vi "Menu Button - Load Config File.vi"(8 "error in (no error)":errorcluster, 11 "Path":path=path "C:/Projects/Trackside-CrawlerFinalDriveTestStand/Codeline/Main Codeline/Software/Config Files_Host/MenuConfig.ini") -> (0 "error out":errorcluster, 1 "Button[]":string[](array[string]), 2 "Level[]":string[](array[string]), 3 "MenuConfig":variant)   [LabVIEW 2019, in "Menu Button.xctl"]
doc: "JSMA Module Template - Top Level UI 0.2.0.4\nRob Humfeld - Jet Engineering\nCopyright (c) 2019, Jet Engineering"
uses:
  Menu Button.xctl
  Button Config Cluster STYP.ctl
  <vilib>/Utility/config.llb/Read Key (String).vi
  <vilib>/Utility/config.llb/Read Key (Boolean).vi
  <vilib>/Utility/config.llb/NI_LVConfig.lvlib
panel:
  out "Color[]":string[](array[string])
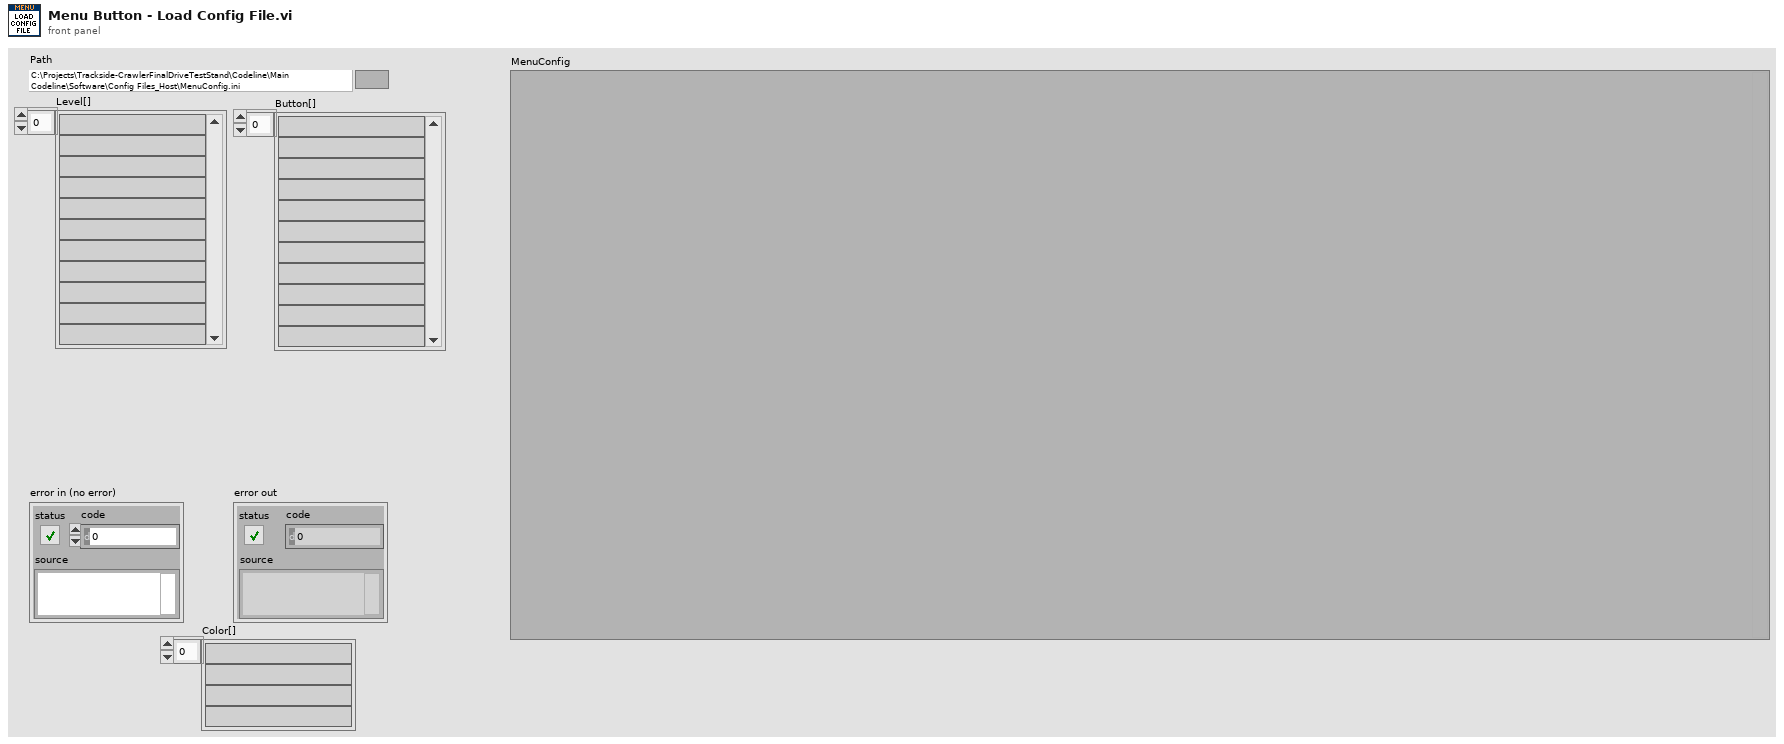
[diagram p1: front panel]
types:
  T1 = typedef "Menu Button.xctl/Button Config Cluster STYP.ctl" = cluster{"ID":string, "Name":string, "Action":string, "Value":string, "Enable?":bool, "Color":string}
  T2 = typedef "NI_LVConfig.lvlib/Config Data RefNum.ctl" = refnum<k1>
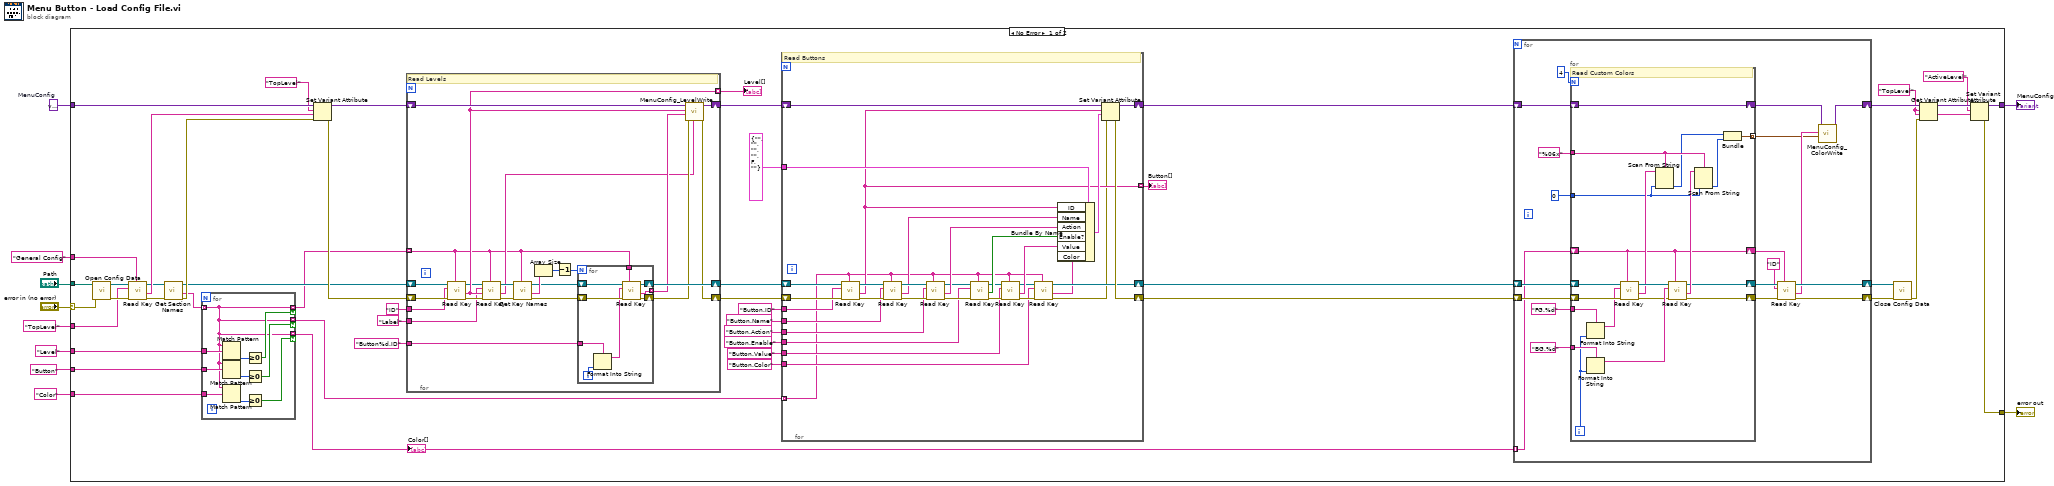
[diagram p0: block diagram]
diagram:
  w7 = variant  # MenuConfig
  n1 = case shown="No Error" "error in (no error)" {
    selector: "error in (no error)" -> [w59 w174]
    tunnel: [w35 w174] -> w9
    tunnel: "Path" -> [w60 _]
    tunnel: w7 -> [w56 w173]
    tunnel: "TopLevel" ("key") -> [w49 _]
    tunnel: "General Config" ("section") -> [w55 _]
    tunnel: [w38 w173] -> w4
    tunnel: "Level" ("key") -> [w28 _]
    tunnel: "Button" ("key") -> [w27 _]
    tunnel: "Color" ("key") -> [w23 _]
    frame No Error {
      w16 = "TopLevel" ("name")
      n2 = call <vilib>:"Open Config Data.vi"("error in (no error)"=w59, "configuration file path"=w60) -> ("error out"=w57:errorcluster, "refnum"=w58:T2)  [unwired: 7 in, 1 out]
      n3 = call-poly <vilib>:"Read Key.vi"("section"=w55, "error in (no error)"=w57, "key"=w49, "refnum"=w58) -> ("error out"=w32:errorcluster, "value"=w54:string, "refnum out"=w33:T2)  [unwired: 4 in, 1 out]
      n4 = call <vilib>:"Get Section Names.vi"("error in (no error)"=w32, "refnum"=w33) -> ("error out"=w31:errorcluster, "section names"=w29:string[], "refnum out"=w30:T2)  [unwired: 7 in]
      n5 = for {
        tunnel: w29 -> [w100] mode=indexing
        tunnel: w28 -> [w109]
        tunnel: w27 -> [w108]
        tunnel: [w100] -> w18 mode=indexing if=w105
        tunnel: [w100] -> w17 mode=indexing if=w104
        tunnel: w23 -> [w103]
        tunnel: [w100] -> w14 mode=indexing if=w101
        n6 = Match Pattern(string=w100, regular expression=w109) -> (offset past match=w107:i32)  [unwired: 1 in, 3 out]
        n7 = Match Pattern(string=w100, regular expression=w108) -> (offset past match=w106:i32)  [unwired: 1 in, 3 out]
        n8 = Match Pattern(string=w100, regular expression=w103) -> (offset past match=w102:i32)  [unwired: 1 in, 3 out]
        n9 = Greater Or Equal To 0?(x=w107) -> (x >= 0?=w105:bool)
        n10 = Greater Or Equal To 0?(x=w106) -> (x >= 0?=w104:bool)
        n11 = Greater Or Equal To 0?(x=w102) -> (x >= 0?=w101:bool)
      }
      "Color[]" <- w14
      n12 = Set Variant Attribute(Variant=w56, name="TopLevel", value=w54, error in=w31) -> (Variant out=w51:variant, error out=w50:errorcluster)  [unwired: 1 out]
      n13 = for {
        shift-right: [w152] -> w47
        shift-left: w50 -> [w162]
        shift-right: [w159] -> w46
        shift-left: w30 -> [w163]
        tunnel: "ID" ("format string") -> [w154]
        tunnel: "Button%d.ID" ("format string") -> [w157]
        shift-right: [w151] -> w41
        shift-left: w51 -> [w155]
        tunnel: [w148] -> w25 mode=indexing
        tunnel: "Label" ("format string") -> [w143]
        tunnel: w18 -> [w141] mode=indexing
        # "Read Levels"
        n14 = call-poly <vilib>:"Read Key.vi"("section"=w141, "error in (no error)"=w162, "key"=w154, "refnum"=w163) -> ("error out"=w147:errorcluster, "value"=w148:string, "refnum out"=w144:T2)  [unwired: 4 in, 1 out]
        n15 = call-poly <vilib>:"Read Key.vi"("section"=w141, "error in (no error)"=w147, "default value"=w148, "key"=w143, "refnum"=w144) -> ("error out"=w146:errorcluster, "value"=w142:string, "refnum out"=w145:T2)  [unwired: 3 in, 1 out]
        n16 = call <vilib>:"Get Key Names.vi"("section"=w141, "error in (no error)"=w146, "refnum"=w145) -> ("error out"=w156:errorcluster, "key names"=w161:string[], "refnum out"=w158:T2)  [unwired: 5 in, 1 out]
        n17 = Array Size(array=w161) -> (size(s)=w160:i32)
        n18 = Decrement(x=w160) -> (x-1=w150:i32)
        n19 = for {
          N: w150 -> [_]
          shift-right: [w169] -> w159
          shift-left: w158 -> [w170]
          tunnel: w157 -> [w172]
          tunnel: w141 -> [w168]
          shift-right: [w166] -> w153
          shift-left: w156 -> [w167]
          tunnel: [w164] -> w149 mode=indexing
          i -> [w171]
          n20 = Format Into String(format string=w172, w171) -> (resulting string=w165:string)  [unwired: 2 in, 1 out]
          n21 = call-poly <vilib>:"Read Key.vi"("section"=w168, "error in (no error)"=w167, "key"=w165, "refnum"=w170) -> ("error out"=w166:errorcluster, "value"=w164:string, "refnum out"=w169:T2)  [unwired: 4 in, 1 out]
        }
        n22 = call "MenuConfig_LevelWrite.vi"("Level.Label (\"\": Same as ID)"=w142, "error in (no error)"=w153, "Button.ID[]"=w149, "Level.ID"=w148, "MenuConfig"=w155) -> ("error out"=w152:errorcluster, "MenuConfig"=w151:variant)  [unwired: 5 in]
      }
      "Level[]" <- w25
      n23 = for {
        shift-right: [w128] -> w12
        shift-left: w47 -> [w139]
        tunnel: "Button.ID" ("format string") -> [w127]
        tunnel: "Button.Name" ("format string") -> [w126]
        tunnel: "Button.Action" ("format string") -> [w125]
        shift-right: [w115] -> w11
        shift-left: w46 -> [w140]
        tunnel: T1 {"ID"="", "Name"="", "Action"="", "Value"="", "Enable?"=FALSE, "Color"=""} ("ButtonConfig") -> [w134]
        shift-right: [w130] -> w13
        shift-left: w41 -> [w131]
        tunnel: "Button.Enable" ("format string") -> [w122]
        tunnel: "Button.Value" ("format string") -> [w118]
        tunnel: [w117] -> w26 mode=indexing
        tunnel: "Button.Color" ("format string") -> [w112]
        tunnel: w17 -> [w110] mode=indexing
        # "Read Buttons"
        n24 = call-poly <vilib>:"Read Key.vi"("section"=w110, "error in (no error)"=w139, "key"=w127, "refnum"=w140) -> ("error out"=w138:errorcluster, "value"=w117:string, "refnum out"=w136:T2)  [unwired: 4 in, 1 out]
        n25 = call-poly <vilib>:"Read Key.vi"("section"=w110, "error in (no error)"=w138, "key"=w126, "refnum"=w136) -> ("error out"=w137:errorcluster, "value"=w133:string, "refnum out"=w135:T2)  [unwired: 4 in, 1 out]
        n26 = call-poly <vilib>:"Read Key.vi"("section"=w110, "error in (no error)"=w137, "key"=w125, "refnum"=w135) -> ("error out"=w123:errorcluster, "value"=w132:string, "refnum out"=w124:T2)  [unwired: 4 in, 1 out]
        n27 = call-poly <vilib>:"Read Key.vi"("section"=w110, "error in (no error)"=w123, "key"=w122, "refnum"=w124) -> ("error out"=w119:errorcluster, "value"=w121:bool, "refnum out"=w120:T2)  [unwired: 4 in, 1 out]
        n28 = call-poly <vilib>:"Read Key.vi"("section"=w110, "error in (no error)"=w119, "key"=w118, "refnum"=w120) -> ("error out"=w114:errorcluster, "value"=w116:string, "refnum out"=w115:T2)  [unwired: 4 in, 1 out]
        n29 = call-poly <vilib>:"Read Key.vi"("section"=w110, "error in (no error)"=w114, "key"=w112, "refnum"=w115) -> ("error out"=w113:errorcluster, "value"=w111:string)  [unwired: 4 in, 2 out]
        n30 = Bundle By Name(cluster=w134, "ID"=w117, "Name"=w133, "Action"=w132, "Enable?"=w121, "Value"=w116, "Color"=w111) -> (w129:T1)
        n31 = Set Variant Attribute(Variant=w131, name=w117, value=w129, error in=w113) -> (Variant out=w130:variant, error out=w128:errorcluster)  [unwired: 1 out]
      }
      "Button[]" <- w26
      n32 = for {
        shift-right: [w62] -> w20
        shift-left: w12 -> [w74]
        shift-right: [w65] -> w21
        shift-left: w13 -> [w73]
        shift-right: [w67] -> w22
        shift-left: w11 -> [w72]
        tunnel: w14 -> [w61] mode=indexing
        n33 = for {
          N: 4 -> [_]
          shift-right: [w81] -> w69
          shift-left: w74 -> [w99]
          shift-right: [w82] -> w70
          shift-left: w72 -> [w84]
          shift-right: [w97] -> w66
          shift-left: w73 -> [w97]
          tunnel: "FG.%d" ("format string") -> [w96]
          tunnel: "BG.%d" ("format string") -> [w94]
          tunnel: "%06x" ("format string") -> [w90]
          tunnel: u32 0 -> [w88]
          tunnel: [w85] -> w63 mode=indexing
          shift-right: [w80] -> w71
          shift-left: w61 -> [w80]
          i -> [w93]
          # "Read Custom Colors"
          n34 = Format Into String(format string=w96, w93) -> (resulting string=w95:string)  [unwired: 2 in, 1 out]
          n35 = Format Into String(format string=w94, w93) -> (resulting string=w92:string)  [unwired: 2 in, 1 out]
          n36 = call-poly <vilib>:"Read Key.vi"("section"=w80, "error in (no error)"=w99, "key"=w95, "refnum"=w84) -> ("error out"=w83:errorcluster, "value"=w91:string, "refnum out"=w98:T2)  [unwired: 4 in, 1 out]
          n37 = Scan From String(format string=w90, input string=w91, default 1=w88) -> (output 1=w87:u32)  [unwired: 2 in, 3 out]
          n38 = call-poly <vilib>:"Read Key.vi"("section"=w80, "error in (no error)"=w83, "key"=w92, "refnum"=w98) -> ("error out"=w81:errorcluster, "value"=w89:string, "refnum out"=w82:T2)  [unwired: 4 in, 1 out]
          n39 = Scan From String(format string=w90, input string=w89, default 1=w88) -> (output 1=w86:u32)  [unwired: 2 in, 3 out]
          n40 = Bundle(w87, w86) -> (w85:cluster{u32, u32})  [unwired: 1 in]
        }
        n41 = call-poly <vilib>:"Read Key.vi"("section"=w71, "error in (no error)"=w69, "key"="ID" ("format string"), "refnum"=w70) -> ("error out"=w62:errorcluster, "value"=w64:string, "refnum out"=w67:T2)  [unwired: 4 in, 1 out]
        n42 = call "MenuConfig_ColorWrite.vi"("Colors[4]"=w63, "Color.Name (\"Default\")"=w64, "MenuConfig"=w66) -> ("MenuConfig"=w65:variant)  [unwired: 7 in, 1 out]
      }
      n43 = call <vilib>:"Close Config Data.vi"("error in (no error)"=w20, "refnum"=w22) -> ("error out"=w36:errorcluster)  [unwired: 8 in, 1 out]
      n44 = Get Variant Attribute(Variant=w21, name=w16, default value (empty Variant)=w16, error in=w36) -> (duplicate Variant=w39:variant, value=w15:string)  [unwired: 2 out]
      n45 = Set Variant Attribute(Variant=w39, name="ActiveLevel", value=w15) -> (Variant out=w38:variant, error out=w35:errorcluster)  [unwired: 1 in, 1 out]
    }
    frame Error {
    }
  }
  "error out" <- w9
  "MenuConfig" <- w4
